vi "Get zero move.vi"(8 "error in (no error)":errorcluster, 10 "Current position":cluster{"M1":dbl, "M2 ":dbl}, 11 "Zero position":cluster{"M1":dbl, "M2":dbl}={"M1"=60.0, "M2"=30.0}) -> (0 "error out":errorcluster, 3 "Cluster out":T1={"Timeout"=0, "Max angle"=0.0, "Zero position"={"M1"=60.0, "M2"=30.0}, "Position params"={"Motor"=enum."All", "Direction M1"=enum."CW", "Direction M2"=enum."CW", "Acquiring?"=FALSE, "Position0"={"M1 pos"=0.0, "M2 pos "=0.0}, "Last Position"={"M1 pos"=0.0, "M2 pos "=0.0}, "Steps"=0, "Module ID"=0}})   [LabVIEW 2020]
doc: "Calcualtes motor maximum steps from the expected displacement of both motors, creates the Acquisition arguments cluster from the movement inputs."
uses:
  controls/Motor direction ---typedef.ctl
  controls/Move to zero ---argument.ctl
  controls/Position arguments ---typedef.ctl
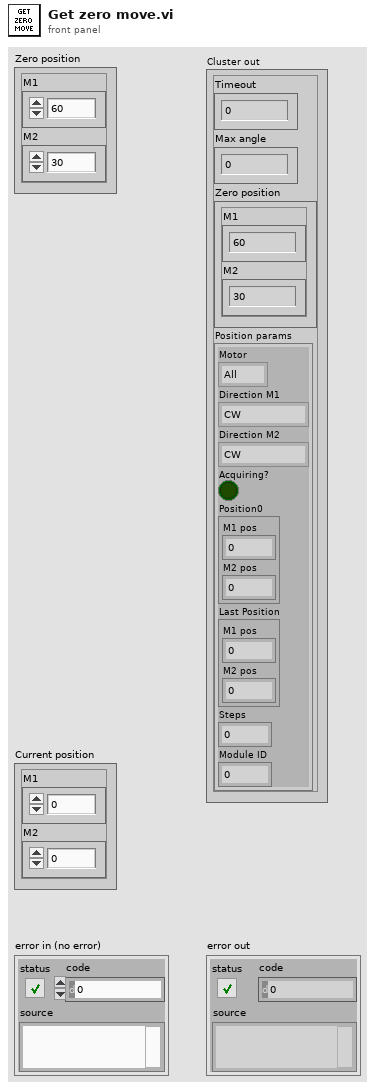
[diagram p1: front panel]
types:
  T1 = typedef "Move to zero ---argument.ctl" = cluster{"Timeout":i32, "Max angle":dbl, "Zero position":cluster{"M1":dbl, "M2":dbl}, "Position params":T2}
  T2 = typedef "Position arguments ---typedef.ctl" = cluster{"Motor":enum16{"All", "M1", "M2"}, "Direction M1":T3, "Direction M2":T3, "Acquiring?":bool, "Position0":cluster{"M1 pos":dbl, "M2 pos ":dbl}, "Last Position":cluster{"M1 pos":dbl, "M2 pos ":dbl}, "Steps":i32, "Module ID":i32}
  T3 = typedef "Motor direction ---typedef.ctl" = enum16{"CW", "CCW", "IDLE"}
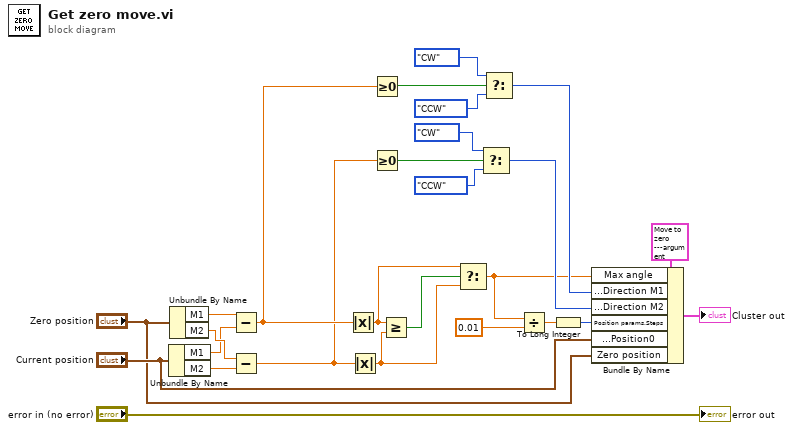
[diagram p0: block diagram]
diagram:
  n1 = Unbundle By Name("Current position") -> ("M1"=w24:dbl, "M2"=w26:dbl)
  n2 = Unbundle By Name("Zero position") -> ("M1"=w23:dbl, "M2"=w25:dbl)
  n3 = Subtract(x=w23, y=w24) -> (x-y=w19:dbl)
  n4 = Subtract(x=w25, y=w26) -> (x-y=w18:dbl)
  n5 = Absolute Value(x=w19) -> (abs(x)=w6:dbl)
  n6 = Absolute Value(x=w18) -> (abs(x)=w5:dbl)
  n7 = Greater Or Equal To 0?(x=w19) -> (x >= 0?=w17:bool)
  n8 = Greater Or Equal To 0?(x=w18) -> (x >= 0?=w12:bool)
  n9 = Greater Or Equal?(x=w6, y=w5) -> (x >= y?=w7:bool)
  n10 = Select(t=w6, s=w7, f=w5) -> (s? t:f=w4:dbl)
  n11 = Select(t=Motor_direction_---typedef."CW" ("Direction M1"), s=w12, f=Motor_direction_---typedef."CCW") -> (s? t:f=w10:T3)
  n12 = Select(t=Motor_direction_---typedef."CW" ("Direction M1"), s=w17, f=Motor_direction_---typedef."CCW") -> (s? t:f=w11:T3)
  n13 = Divide(x=w4, y=0.01) -> (x/y=w2:dbl)
  n14 = To Long Integer(number=w2) -> (32bit integer=w1:i32)
  n15 = Bundle By Name(cluster=T1 {"Timeout"=0, "Max angle"=0.0, "Zero position"={"M1"=60.0, "M2"=30.0}, "Position params"={"Motor"=enum."All", "Direction M1"=enum."CW", "Direction M2"=enum."CW", "Acquiring?"=FALSE, "Position0"={"M1 pos"=0.0, "M2 pos "=0.0}, "Last Position"={"M1 pos"=0.0, "M2 pos "=0.0}, "Steps"=0, "Module ID"=0}} ("Cluster out"), "Max angle"=w4, "Position params.Direction M1"=w11, "Position params.Direction M2"=w10, "Position params.Steps"=w1, "Position params.Position0"="Current position", "Zero position"="Zero position") -> (→"Cluster out":T1)
  "error out" <- "error in (no error)"
